vi "ECS-100X-FPGA1-EPTx.vi"() -> ()   [LabVIEW 2015, in "ECS-FPGA.lvlib"]
uses:
  ECS-FPGA.lvlib
  <vilib>/addons/Combustion Analysis System/FPGA/Controls/CAS - FPGA - Sample Data.ctl
  <vilib>/addons/Combustion Analysis System/FPGA/Controls/CAS - FPGA - EPT Data.ctl
  <vilib>/addons/Combustion Analysis System/FPGA/Controls/CAS - FPGA - Encoder Signals.ctl
  <vilib>/addons/Combustion Analysis System/FPGA/Controls/CAS - FPGA - Sample Control.ctl
  <vilib>/addons/Combustion Analysis System/FPGA/Controls/CAS - FPGA - Encoder Settings.ctl
  <vilib>/addons/Combustion Analysis System/FPGA/Controls/CAS - FPGA - EPT Control.ctl
  <vilib>/Powertrain Controls/Device Drivers/Engine Position Tracking/EPTx/RevA/FPGA/Controls/EPTxSupervisor.ctl
  <vilib>/Powertrain Controls/Device Drivers/Engine Position Tracking/EPTx/RevA/FPGA/Controls/EPTxConfig.ctl
  <vilib>/Powertrain Controls/Device Drivers/Engine Position Tracking/EPTx/RevA/FPGA/Controls/EPTxControl.ctl
  <vilib>/Powertrain Controls/Device Drivers/Engine Position Tracking/EPTx/RevA/FPGA/Controls/EPTxTooth.ctl
  <vilib>/Powertrain Controls/Device Drivers/Engine Position Tracking/EPTx/RevA/FPGA/Controls/EPTxEncoderConfig.ctl
  <vilib>/Powertrain Controls/Device Drivers/Engine Position Tracking/EPTx/RevA/FPGA/Controls/EPTxAAPControl.ctl
  <vilib>/Powertrain Controls/Device Drivers/Engine Position Tracking/EPTx/RevA/FPGA/Controls/EPTxFuelSparkControl.ctl
  <vilib>/Powertrain Controls/Device Drivers/FPGA Knock/RevA/FPGA/Controls/Knock Settings.ctl
  <vilib>/Powertrain Controls/Device Drivers/FPGA Knock/RevA/FPGA/Controls/EPTx Window.ctl
  <vilib>/Platform/TimedLoop/XDataNode/timing_clust.ctl
  <vilib>/Platform/TimedLoop/XDataNode/nitl_modes.ctl
  <vilib>/Platform/TimedLoop/XDataNode/wakeup.ctl
  <vilib>/Powertrain Controls/Device Drivers/Engine Position Tracking/EPTx/RevA/FPGA/Controls/EPTxSignals.ctl
  <vilib>/rvi/Emulation/niFpgaGetClockAttributes.vi
  <vilib>/rvi/Emulation/niFpgaSctlEmulationGetInTimedLoop.vi
  <vilib>/rvi/Emulation/niFpgaEmulationReportErrorSimple.vi
  <vilib>/rvi/eio/common/nirviEmuTemplateMethod_errors.vi
  <vilib>/rvi/Emulation/niFpgaCriticalErrorInLSC.vi
  <vilib>/rvi/Emulation/niFpgaProcessEmulError.vi
  <vilib>/eio/EIOMethodNode/EIOMethodNode.xnode
  <vilib>/eio/EIONode/EIONode.xnode
  <vilib>/LabVIEW Targets/FPGA/RIO/nicrio_985x_controls.llb/CAN_IO_Frame Cluster.ctl
  <vilib>/LabVIEW Targets/FPGA/RIO/nicrio_985x_controls.llb/CAN_IO_Frame Type.ctl
  <vilib>/Platform/TimedLoop/XDataNode/XDataNode.xnode
  <vilib>/Platform/TimedLoop/XDataNode/XDNodeRunTimeDep.lvlib
  <vilib>/Powertrain Controls/Device Drivers/Engine Position Tracking/EPTx/RevA/FPGA/EPTx - RevA - FPGA.lvlib
  <vilib>/Powertrain Controls/Device Drivers/FPGA Knock/RevA/FPGA/Knock - RevA - FPGA.lvlib
panel:
  in  "Knock.SensorIndexes":i32[](array[numeric])=[0, 0, 0, 0, 0, 0, 0, 0, 0, 0, 0, 0, 0, 0, 0, 0]
  out "Knock.Running":bool
  in  "Knock.Windows":cluster{"Index":fxp<+,4,4>, "EPT Windows":T1}
  in  "Knock.Settings":T2={"Sample Clock [Ticks]"=0, "Threshold"=0.0, "Coeff A"=[0.0, 0.0, 0.0, 0.0], "Coeff B"=[0.0, 0.0, 0.0, 0.0, 0.0, 0.0]}
  out "Knock.Results":bool[](array[boolean])
  out "Knock.Intensity":fxp<+,8,4>[](array[numeric]) format="%.6g"
  in  "O2-1.Control":T3
  out "O2-1.Data":T4
  in  "DI-1.PlsGen_Config_Channel3":T5
  in  "DI-1.PlsGen_Config_Channel2":T5
  in  "DI-1.PlsGen_Config_Channel1":T5
  in  "EPTx.Gate/Reset":u8=1
  in  "EPTx.EncoderZ":u8=1
  in  "EPTx.EncoderB":u8=1
  in  "EPTx.EncSignalSelect":bool
  in  "ESTTL-1.Sequences":T6(array[cluster])
  in  "ESTTL-1.Config":T7
  in  "PFI-1.FuelControl 4":T8
  in  "PFI-1.FuelControl 3":T8
  in  "PFI-1.FuelControl 2":T8
  in  "PFI-1.FuelControl 1":T8
  out "EPTx.Aux4CaptureCAD":fxp<+,18,11>
  out "EPTx.Aux3CaptureCAD":fxp<+,18,11>
  out "EPTx.Aux2CaptureCAD":fxp<+,18,11>
  out "EPTx.Aux1CaptureCAD":fxp<+,18,11>
  out "EPTx.Aux4EdgeCount":u8
  out "EPTx.Aux3EdgeCount":u8
  out "EPTx.Aux2EdgeCount":u8
  out "EPTx.Aux1EdgeCount":u8
  in  "EPTx.Aux4AngleCapture":T9
  in  "EPTx.Aux3AngleCapture":T9
  in  "EPTx.Aux2AngleCapture":T9
  in  "EPTx.Aux1AngleCapture":T9
  in  "EPTx.EncoderA":u8=1
  in  "EPTxEncoderConfig":T10
  out "EPTxTooth":T11
  in  "EPTxControl":T12
  in  "EPTxConfig":T13
  out "EPTxSupervisor":T14
  out "ADCombo-1.DigitalTriggers":u32
  in  "UserData.Data0":u32
  in  "UserData.Data1":u32
  in  "UserData.Data2":u32
  in  "UserData.Data3":u32
  in  "UserData.Period [ms]":u32=1
  in  "UserData.EnableFPGAData":bool
  in  "UserData.Data4":u32
  in  "UserData.Data5":u32
  in  "UserData.Data6":u32
  in  "UserData.Data7":u32
  in  "CAS-EPT Control":T15
  in  "CAS-Encoder Settings":T16
  in  "CAS-Sample Control":T17
  out "CAS-Encoder Signals":T18
  out "CAS-EPT Data":T19
  out "CAS-Sample Data":T20
  in  "CAS-Encoder Debug":bool
  out "CAS-Debug Overflow":bool
  out "Throttle-1.Data":T21 caption="ThrottleData"
  in  "Throttle-1.Control":T22 caption="ThrottleControl"
  out "ADCombo-1.VRHallData":T23 caption="VRHallData"
  in  "EPTx.Aux4":u8=2
  in  "EPTx.Aux2":u8=1
  out "DI-1.Data":T24 caption="DIData"
  in  "ADCombo-1.VRHallInvert":u8
  in  "ADCombo-1.VR1.Filt":u16
  in  "ADCombo-1.VR2.Filt":u16
  in  "ADCombo-1.Hall1.Filt":u16
  in  "ADCombo-1.Hall2.Filt":u16
  in  "9411-1.0.Filt":u16
  in  "9411-1.1.Filt":u16
  in  "9411-1.2.Filt":u16
  in  "9411-1.3.Filt":u16
  in  "9411-1.4.Filt":u16
  in  "9411-1.5.Filt":u16
  in  "9411-1.Invert":u8
  in  "9755-1.Sensor 1 Enable":bool
  in  "9755-1.RxID 1":u32=418385746 format="%08x"
  in  "9755-1.TxID":u32=419356416 format="%08x"
  in  "9755-1.CAN0 Restart":bool
  out "9755-1.NOxSensorData 1":T25={"NOx (bits)"=0, "O2 (bits)"=0, "Sensor Supply Status"=3, "Sensor Temperature Status"=12, "NOx Signal Status"=48, "O2 Signal Status"=192, "Heater Mode Status"=96, "Heater Circuit Status"=31, "NOx Circuit Status"=31, "O2 Circuit Status"=31, "NOx Sensor Module Present"=FALSE} {"Heater Mode Status" items=["AUTO MODE"=0, "HEATUP SLOPE 3 OR 4"=32, "HEATUP SLOPE 1 OR 2"=64, "HEATER OFF / PREHEAT"=96]; "O2 Circuit Status" items=["OPEN WIRE"=3, "SHORT CIRCUIT"=5, "NO ERROR"=31]; "NOx Circuit Status" items=["OPEN WIRE"=3, "SHORT CIRCUIT"=5, "NO ERROR"=31]; "Heater Circuit Status" items=["OPEN WIRE"=3, "SHORT CIRCUIT"=5, "NO ERROR"=31]; "Sensor Temperature Status" items=["NOT AT TEMPERATURE"=0, "AT TEMPERATURE"=4, "ERROR"=8, "NOT AVAILABLE"=12]; "O2 Signal Status" items=["NOT VALID"=0, "VALID"=64, "ERROR"=128, "NOT AVAILABLE"=192]; "NOx Signal Status" items=["NOT VALID"=0, "VALID"=16, "ERROR"=32, "NOT AVAILABLE"=48]; "Sensor Supply Status" items=["NOT IN RANGE", "SUPPLY IN RANGE", "ERROR", "NOT AVAILABLE"]}
  out "9755-1.RxID Actual":u32 format="%08x"
  in  "9755-1.Sensor 2 Enable":bool
  in  "9755-1.RxID 2":u32=418385489 format="%08x"
  out "9755-1.NOxSensorData 2":T25={"NOx (bits)"=0, "O2 (bits)"=0, "Sensor Supply Status"=3, "Sensor Temperature Status"=12, "NOx Signal Status"=48, "O2 Signal Status"=192, "Heater Mode Status"=96, "Heater Circuit Status"=31, "NOx Circuit Status"=31, "O2 Circuit Status"=31, "NOx Sensor Module Present"=FALSE} {"Heater Mode Status" items=["AUTO MODE"=0, "HEATUP SLOPE 3 OR 4"=32, "HEATUP SLOPE 1 OR 2"=64, "HEATER OFF / PREHEAT"=96]; "O2 Circuit Status" items=["OPEN WIRE"=3, "SHORT CIRCUIT"=5, "NO ERROR"=31]; "NOx Circuit Status" items=["OPEN WIRE"=3, "SHORT CIRCUIT"=5, "NO ERROR"=31]; "Heater Circuit Status" items=["OPEN WIRE"=3, "SHORT CIRCUIT"=5, "NO ERROR"=31]; "Sensor Temperature Status" items=["NOT AT TEMPERATURE"=0, "AT TEMPERATURE"=4, "ERROR"=8, "NOT AVAILABLE"=12]; "O2 Signal Status" items=["NOT VALID"=0, "VALID"=64, "ERROR"=128, "NOT AVAILABLE"=192]; "NOx Signal Status" items=["NOT VALID"=0, "VALID"=16, "ERROR"=32, "NOT AVAILABLE"=48]; "Sensor Supply Status" items=["NOT IN RANGE", "SUPPLY IN RANGE", "ERROR", "NOT AVAILABLE"]}
  in  "Power.TDK_Rly_Ctrl":bool
  in  "Power.12V_Rly_Ctrl":bool
  in  "Power.5V_Rly_Ctrl":bool
  out "ADCombo-1.ModulePresent":bool caption="ModulePresent"
  out "PFI-1.Data":T26 caption="PFIData"
  in  "PFI-1.IPhaseInterface":T27(array[cluster])=[{"IPhaseCurrent"=0, "IPhaseDuration"=0}, {"IPhaseCurrent"=0, "IPhaseDuration"=0}, {"IPhaseCurrent"=0, "IPhaseDuration"=0}, {"IPhaseCurrent"=0, "IPhaseDuration"=0}, {"IPhaseCurrent"=0, "IPhaseDuration"=0}, {"IPhaseCurrent"=0, "IPhaseDuration"=0}, {"IPhaseCurrent"=0, "IPhaseDuration"=0}, {"IPhaseCurrent"=0, "IPhaseDuration"=0}] caption="IPhaseInterface"
  in  "PFI-1.LowsidePWM":T28 caption="LowsidePWM"
  in  "PFI-1.Control":T29 caption="PFIControl"
  out "DI-1.ScopeData":T30 caption="DIScopeData"
  in  "DI-1.ScopeRead":bool caption="DIScopeRead"
  in  "DI-1.IPhaseInterface":T31(array[cluster]) caption="IPhaseInterface"
  in  "DI-1.Control":T32 caption="DIControl"
  in  "EPTx.Aux3":u8
  in  "EPTx.Primary":u8
  in  "EPTx.Aux1":u8
  out "ADCombo-1.Hall1.PPWData":T33
  out "ADCombo-1.Hall2.PPWData":T33
  out "ADCombo-1.VR2.PPWData":T33
  out "ADCombo-1.VR1.PPWData":T33
  out "9411-1.0.PPWData":T33
  out "9411-1.1.PPWData":T33
  out "9411-1.2.PPWData":T33
  out "9411-1.3.PPWData":T33
  out "9411-1.4.PPWData":T33
  out "9411-1.5.PPWData":T33
  out "9411-1.DigitalTriggers":u32
  out "ADCombo-1.AnalogData":T34 caption="AnalogData"
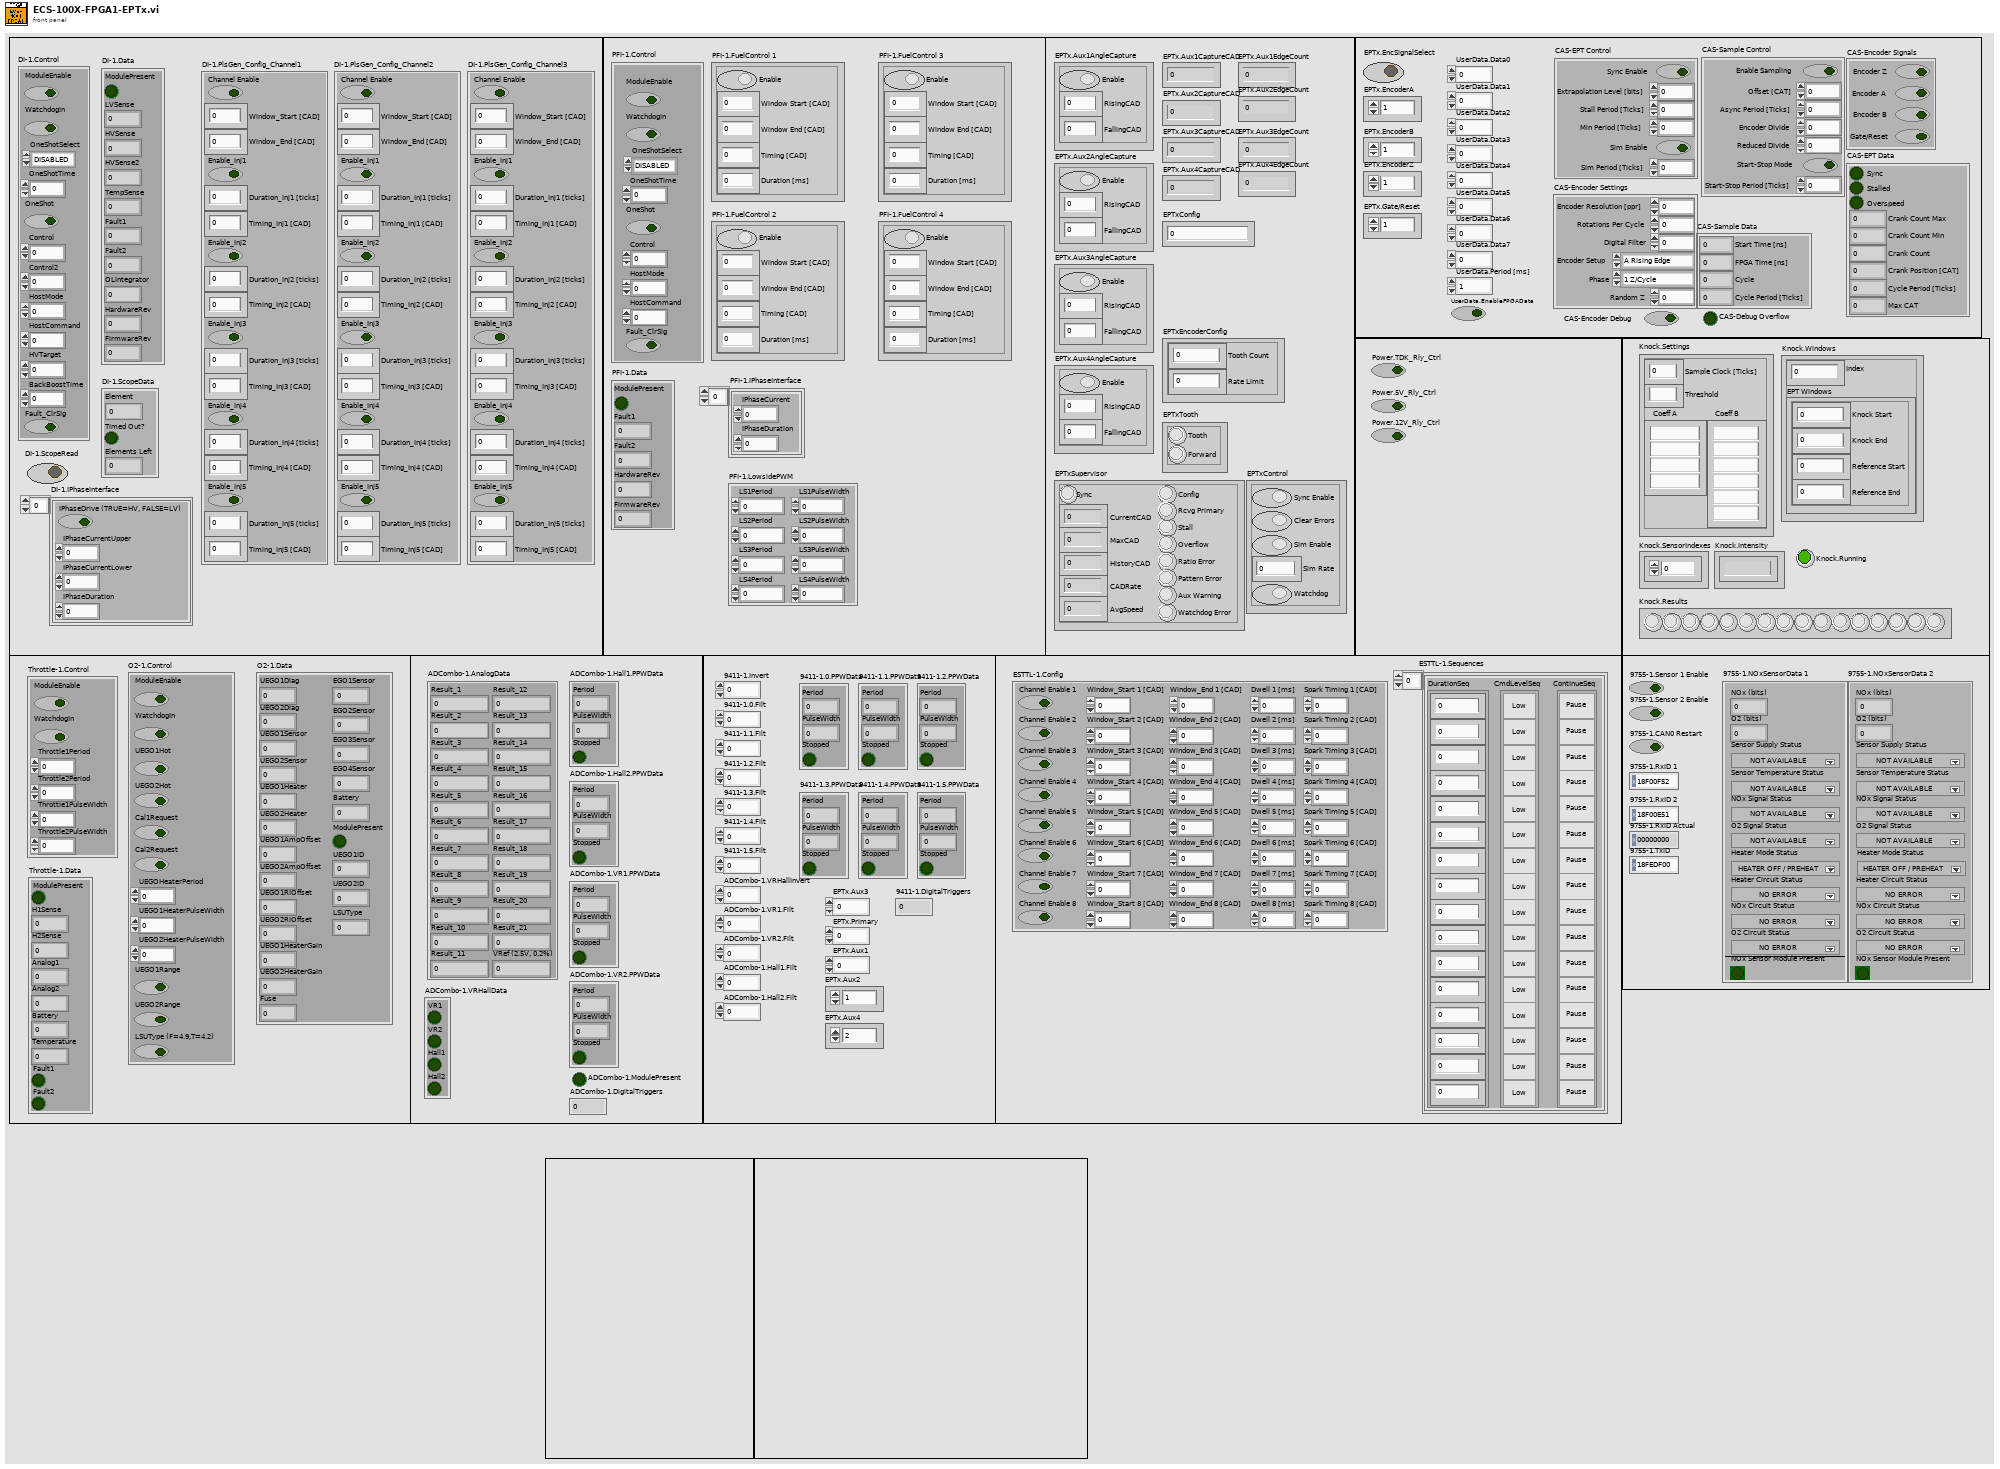
[diagram p1: front panel]
types:
  T1 = typedef "Knock - RevA - FPGA.lvlib/EPTx Window.ctl" = cluster{"Knock Start":fxp<+,18,11>, "Knock End":fxp<+,18,11>, "Reference Start":fxp<+,18,11>, "Reference End":fxp<+,18,11>}
  T2 = typedef "Knock - RevA - FPGA.lvlib/Knock Settings.ctl" = cluster{"Sample Clock [Ticks]":u16, "Threshold":fxp<+,10,4>, "Coeff A":fxp<+/-,16,2>[], "Coeff B":fxp<+/-,20,3>[]}
  T3 = cluster{"ModuleEnable":bool, "WatchdogIn":bool, "UEGO1Hot":bool, "UEGO2Hot":bool, "Cal1Request":bool, "Cal2Request":bool, "UEGOHeaterPeriod":u16, "UEGO1HeaterPulseWidth":u16, "UEGO2HeaterPulseWidth":u16, "UEGO1Range":bool, "UEGO2Range":bool, "LSUType (F=4.9,T=4.2)":bool}
  T4 = cluster{"UEGO1Diag":u8, "UEGO2Diag":u8, "UEGO1Sensor":u16, "UEGO2Sensor":u16, "UEGO1Heater":u16, "UEGO2Heater":u16, "UEGO1AmpOffset":u16, "UEGO2AmpOffset":u16, "UEGO1RIOffset":u16, "UEGO2RIOffset":u16, "UEGO1HeaterGain":u16, "UEGO2HeaterGain":u16, "Fuse":u16, "EGO1Sensor":u16, "EGO2Sensor":u16, "EGO3Sensor":u16, "EGO4Sensor":u16, "Battery":u16, "ModulePresent":bool, "UEGO1ID":u8, "UEGO2ID":u8, "LSUType":u8}
  T5 = cluster{"Channel Enable":bool, "Window_Start [CAD]":fxp<+,18,11>, "Window_End [CAD]":fxp<+,18,11>, "Enable_Inj1":bool, "Duration_Inj1 [ticks]":u32, "Timing_Inj1 [CAD]":fxp<+,18,11>, "Enable_Inj2":bool, "Duration_Inj2 [ticks]":u32, "Timing_Inj2 [CAD]":fxp<+,18,11>, "Enable_Inj3":bool, "Duration_Inj3 [ticks]":u32, "Timing_Inj3 [CAD]":fxp<+,18,11>, "Enable_Inj4":bool, "Duration_Inj4 [ticks]":u32, "Timing_Inj4 [CAD]":fxp<+,18,11>, "Enable_Inj5":bool, "Duration_Inj5 [ticks]":u32, "Timing_Inj5 [CAD]":fxp<+,18,11>}
  T6 = cluster{"DurationSeq":u32[], "CmdLevelSeq":bool[], "ContinueSeq":bool[]}[]
  T7 = cluster{"Channel Enable 1":bool, "Window_Start 1 [CAD]":fxp<+,18,11>, "Window_End 1 [CAD]":fxp<+,18,11>, "Dwell 1 [ms]":fxp<+/-,22,9>, "Spark Timing 1 [CAD]":fxp<+,18,11>, "Channel Enable 2":bool, "Window_Start 2 [CAD]":fxp<+,18,11>, "Window_End 2 [CAD]":fxp<+,18,11>, "Dwell 2 [ms]":fxp<+/-,22,9>, "Spark Timing 2 [CAD]":fxp<+,18,11>, "Channel Enable 3":bool, "Window_Start 3 [CAD]":fxp<+,18,11>, "Window_End 3 [CAD]":fxp<+,18,11>, "Dwell 3 [ms]":fxp<+/-,22,9>, "Spark Timing 3 [CAD]":fxp<+,18,11>, "Channel Enable 4":bool, "Window_Start 4 [CAD]":fxp<+,18,11>, "Window_End 4 [CAD]":fxp<+,18,11>, "Dwell 4 [ms]":fxp<+/-,22,9>, "Spark Timing 4 [CAD]":fxp<+,18,11>, "Channel Enable 5":bool, "Window_Start 5 [CAD]":fxp<+,18,11>, "Window_End 5 [CAD]":fxp<+,18,11>, "Dwell 5 [ms]":fxp<+/-,22,9>, "Spark Timing 5 [CAD]":fxp<+,18,11>, "Channel Enable 6":bool, "Window_Start 6 [CAD]":fxp<+,18,11>, "Window_End 6 [CAD]":fxp<+,18,11>, "Dwell 6 [ms]":fxp<+/-,22,9>, "Spark Timing 6 [CAD]":fxp<+,18,11>, "Channel Enable 7":bool, "Window_Start 7 [CAD]":fxp<+,18,11>, "Window_End 7 [CAD]":fxp<+,18,11>, "Dwell 7 [ms]":fxp<+/-,22,9>, "Spark Timing 7 [CAD]":fxp<+,18,11>, "Channel Enable 8":bool, "Window_Start 8 [CAD]":fxp<+,18,11>, "Window_End 8 [CAD]":fxp<+,18,11>, "Dwell 8 [ms]":fxp<+/-,22,9>, "Spark Timing 8 [CAD]":fxp<+,18,11>}
  T8 = typedef "EPTx - RevA - FPGA.lvlib/EPTxFuelSparkControl.ctl" = cluster{"Enable":bool, "Window Start [CAD]":fxp<+,18,11>, "Window End [CAD]":fxp<+,18,11>, "Timing [CAD]":fxp<+,18,11>, "Duration [ms]":fxp<+/-,22,9>}
  T9 = typedef "EPTx - RevA - FPGA.lvlib/EPTxAAPControl.ctl" = cluster{"Enable":bool, "RisingCAD":fxp<+,18,11>, "FallingCAD":fxp<+,18,11>}
  T10 = typedef "EPTx - RevA - FPGA.lvlib/EPTxEncoderConfig.ctl" = cluster{"Tooth Count":fxp<+,12,12>, "Rate Limit":fxp<+,12,12>}
  T11 = typedef "EPTx - RevA - FPGA.lvlib/EPTxTooth.ctl" = cluster{"Tooth":bool, "Forward":bool}
  T12 = typedef "EPTx - RevA - FPGA.lvlib/EPTxControl.ctl" = cluster{"Sync Enable":bool, "Clear Errors":bool, "Sim Enable":bool, "Sim Rate":fxp<+,24,6>, "Watchdog":bool}
  T13 = typedef "EPTx - RevA - FPGA.lvlib/EPTxConfig.ctl" = u64
  T14 = typedef "EPTx - RevA - FPGA.lvlib/EPTxSupervisor.ctl" = cluster{"Sync":bool, "CurrentCAD":fxp<+,18,11>, "MaxCAD":fxp<+,11,11>, "HistoryCAD":fxp<+,11,11>, "CADRate":fxp<+,22,8>, "AvgSpeed":fxp<+,17,15>, "Config":bool, "Rcvg Primary":bool, "Stall":bool, "Overflow":bool, "Ratio Error":bool, "Pattern Error":bool, "Aux Warning":bool, "Watchdog Error":bool}
  T15 = typedef "CAS - FPGA - EPT Control.ctl" = cluster{"Sync Enable":bool, "Extrapolation Level [bits]":u8, "Stall Period [Ticks]":u32, "Min Period [Ticks]":u32, "Sim Enable":bool, "Sim Period [Ticks]":u32}
  T16 = typedef "CAS - FPGA - Encoder Settings.ctl" = cluster{"Encoder Resolution [ppr]":u16, "Rotations Per Cycle":u8, "Digital Filter":u16, "Encoder Setup":enum8{"A Rising Edge", "A Any Edge", "A & B Any Edge"}, "Phase":enum8{"1 Z/Cycle", "Gate Z", "Random Z", "Reset Z"}, "Random Z":u8}
  T17 = typedef "CAS - FPGA - Sample Control.ctl" = cluster{"Enable Sampling":bool, "Offset [CAT]":i32, "Async Period [Ticks]":u32, "Encoder Divide":u8, "Reduced Divide":u8, "Start-Stop Mode":bool, "Start-Stop Period [Ticks]":u32}
  T18 = typedef "CAS - FPGA - Encoder Signals.ctl" = cluster{"Encoder Z":bool, "Encoder A":bool, "Encoder B":bool, "Gate/Reset":bool}
  T19 = typedef "CAS - FPGA - EPT Data.ctl" = cluster{"Sync":bool, "Stalled":bool, "Overspeed":bool, "Crank Count Max":u16, "Crank Count Min":u16, "Crank Count":u16, "Crank Position [CAT]":u16, "Cycle Period [Ticks]":u32, "Max CAT":u16}
  T20 = typedef "CAS - FPGA - Sample Data.ctl" = cluster{"Start Time [ns]":u64, "FPGA Time [ns]":u64, "Cycle":u32, "Cycle Period [Ticks]":u32}
  T21 = cluster{"ModulePresent":bool, "H1Sense":i16, "H2Sense":i16, "Analog1":i16, "Analog2":i16, "Battery":i16, "Temperature":i16, "Fault1":bool, "Fault2":bool}
  T22 = cluster{"ModuleEnable":bool, "WatchdogIn":bool, "Throttle1Period":u16, "Throttle2Period":u16, "Throttle1PulseWidth":i16, "Throttle2PulseWidth":i16}
  T23 = cluster{"VR1":bool, "VR2":bool, "Hall1":bool, "Hall2":bool}
  T24 = cluster{"ModulePresent":bool, "LVSense":u8, "HVSense":u8, "HVSense2":u8, "TempSense":i8, "Fault1":u8, "Fault2":u8, "OLIntegrator":u32, "HardwareRev":u8, "FirmwareRev":u8}
  T25 = cluster{"NOx (bits)":u16, "O2 (bits)":u16, "Sensor Supply Status":u8, "Sensor Temperature Status":u8, "NOx Signal Status":u8, "O2 Signal Status":u8, "Heater Mode Status":u8, "Heater Circuit Status":u8, "NOx Circuit Status":u8, "O2 Circuit Status":u8, "NOx Sensor Module Present":bool}
  T26 = cluster{"ModulePresent":bool, "Fault1":u8, "Fault2":u8, "HardwareRev":u8, "FirmwareRev":u8}
  T27 = cluster{"IPhaseCurrent":u16, "IPhaseDuration":u16}[]
  T28 = cluster{"LS1Period":u32, "LS1PulseWidth":u32, "LS2Period":u32, "LS2PulseWidth":u32, "LS3Period":u32, "LS3PulseWidth":u32, "LS4Period":u32, "LS4PulseWidth":u32}
  T29 = cluster{"ModuleEnable":bool, "WatchdogIn":bool, "OneShotSelect":enum8{"DISABLED", "PFI 1", "PFI 2", "PFI 3", "PFI 4"}, "OneShotTime":u32, "OneShot":bool, "Control":u16, "HostMode":u8, "HostCommand":u32, "Fault_ClrSig":bool}
  T30 = cluster{"Element":u32, "Timed Out?":bool, "Elements Left":u32}
  T31 = cluster{"IPhaseDrive (TRUE=HV, FALSE=LV)":bool, "IPhaseCurrentUpper":u16, "IPhaseCurrentLower":u16, "IPhaseDuration":u16}[]
  T32 = cluster{"ModuleEnable":bool, "WatchdogIn":bool, "OneShotSelect":enum8{"DISABLED", "CHAN 1", "CHAN 2", "CHAN 3"}, "OneShotTime":u32, "OneShot":bool, "Control":u8, "Control2":u8, "HostMode":u8, "HostCommand":u32, "HVTarget":u8, "BackBoostTime":u8, "Fault_ClrSig":bool}
  T33 = cluster{"Period":u32, "PulseWidth":u32, "Stopped":bool}
  T34 = cluster{"Result_1":u16, "Result_2":u16, "Result_3":u16, "Result_4":u16, "Result_5":u16, "Result_6":u16, "Result_7":u16, "Result_8":u16, "Result_9":u16, "Result_10":u16, "Result_11":u16, "Result_12":u16, "Result_13":u16, "Result_14":u16, "Result_15":u16, "Result_16":u16, "Result_17":u16, "Result_18":u16, "Result_19":u16, "Result_20":u16, "Result_21":u16, "VRef (2.5V, 0.2%)":u16}
  T35 = typedef "XDNodeRunTimeDep.lvlib/timing_clust.ctl" = cluster{"Expected End [f-1]":u64, "Actual End [f-1]":u64, "Finished Late? [f-1]":bool, "Expected End [i-1]":u64, "Actual End [i-1]":u64, "Finished Late? [i-1]":bool, "Expected Start [i]":u64, "Actual Start [i]":u64, "Expected Start [f]":u64, "Actual Start [f]":u64, "Source Name":string, "Structure Name":string, "Period":i64, "Deadline":i64, "Offset":i64, "Start":i64, "Priority":i32, "Timeout":i32, "Mode":T36, "Wakeup Reason":T37, "Error":errorcluster, "Source Type":string, "Secondary Source Type":string, "Global End Time":u64, "Global Start Time":u64, "Frame Duration":u64, "Iteration Duration":u64, "Assigned CPU":i32, "I/O Scan Engine Mode":u32}
  T36 = typedef "XDNodeRunTimeDep.lvlib/nitl_modes.ctl" = enum32{"No Change", "Process missed periods, maintain original phase", "Discard missed periods, maintain original phase", "Process missed periods, ignore original phase", "Discard missed periods, ignore original phase"}
  T37 = typedef "XDNodeRunTimeDep.lvlib/wakeup.ctl" = enum32{"Normal", "Aborted", "Asynchronous wakeup", "Timing source error", "Timed loop error", "Timeout"}
  T38 = typedef "EPTx - RevA - FPGA.lvlib/EPTxSignals.ctl" = cluster{"Primary":bool, "Aux 1":bool, "Aux 2":bool, "Aux 3":bool, "Aux 4":bool}
  T39 = typedef "EPTx - RevA - FPGA.lvlib/Encoder.ctl" = cluster{"Encoder A":bool, "Encoder B":bool, "Encoder Z":bool, "Encoder Cam":bool}
  T40 = typedef "CAS - FPGA - Trigger Signals.ctl" = cluster{"Start Trigger (TRIG0)":bool, "Sync Clock (TRIG1)":bool, "Async Clock (TRIG2)":bool, "Sync Data (TRIG3)":bool, "Async Data (TRIG4)":bool, "Reduced Resolution (TRIG5)":bool, "Reserved (TRIG6)":bool, "20MHz Clock (TRIG7)":bool}
  T41 = cluster{"CmdOut1":bool, "CmdOut2":bool, "CmdOut3":bool, "CmdOut4":bool, "CmdOut5":bool, "CmdOut6":bool, "CmdOut7":bool, "CmdOut8":bool}
  T42 = typedef "CAN_IO_Frame Cluster.ctl" = cluster{"timestamp high":u32, "timestamp low":u32, "identifier":u32, "type":T43, "info A":u8, "info B":u8, "data length":u8, "data":u8[]}
  T43 = typedef "CAN_IO_Frame Type.ctl" = enum8{"Data Frame", "Remote Frame", "(reserved)", "(reserved) ", "(reserved)  ", "(reserved)   ", "Bus Error", "Transceiver Fault"}
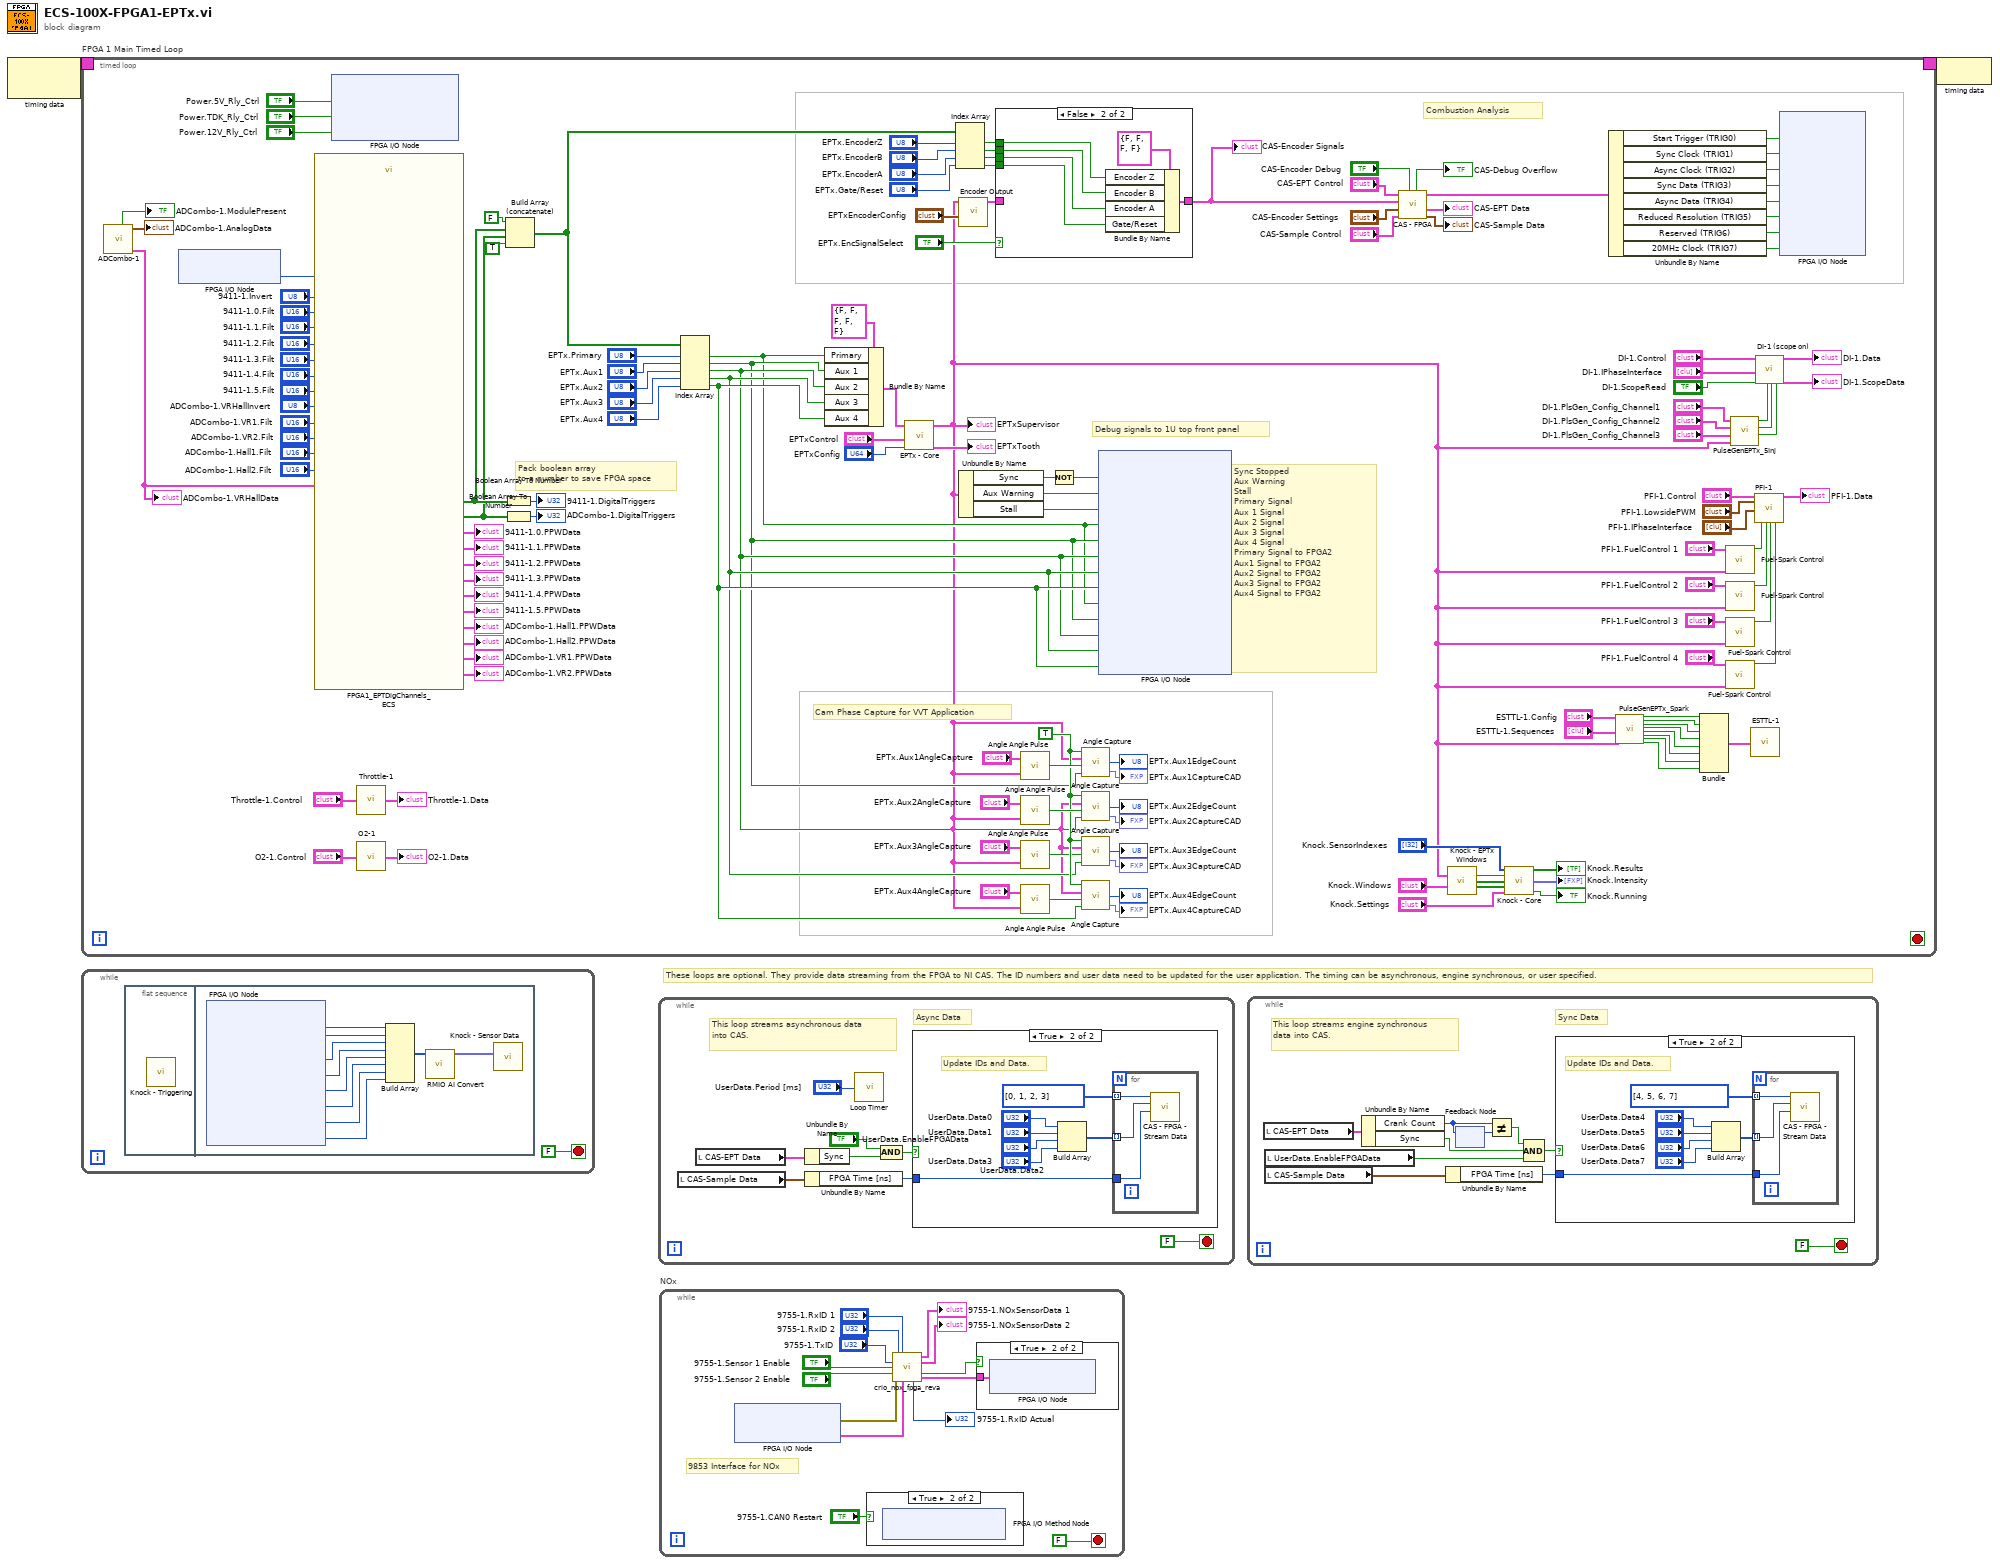
[diagram p0: block diagram]
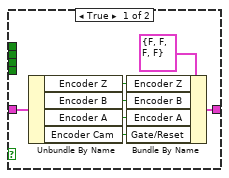
[diagram p6: hidden frame]
diagram:
  # "These loops are optional. They provide data streaming from the FPGA to NI CAS. The ID numbers and user data need to be updated for the user application. The timing can be asynchronous, engine synchronous, or user specified."
  n1 = node-c288() -> (w2:T35)  [unwired: 1 in]
  n2 = timed-loop "FPGA 1 Main Timed Loop" {
    timing: w2 -> [_]
    timing-out: [_] -> w1
    stop <- _ stop-if-true
    w53 = TRUE ("Enable")
    # "Pack boolean array\nto a number to save FPGA space"
    # "Cam Phase Capture for VVT Application"
    # "Combustion Analysis"
    # "Debug signals to 1U top front panel"
    # "Sync Stopped\nAux Warning\nStall\nPrimary Signal\nAux 1 Signal\nAux 2 Signal\nAux 3 Signal\nAux 4 Signal\nPrimary Signal to FPGA2\nAux1 Signal to FPGA2\nAux2 Signal to FPGA2\nAux3 Signal to FPGA2\nAux4 Signal to FPGA2"
    n3 = call "ADCombo-1"() -> ("ADCombo-1_VRHallData"=w150:T23, "ADCombo-1_AnalogData"=→"ADCombo-1.AnalogData":T34, "ADCombo-1_ModulePresent"=→"ADCombo-1.ModulePresent":bool)  [unwired: 5 in, 2 out]
    "ADCombo-1.VRHallData" <- w150
    n4 = xnode "FPGA I/O Node"() -> ("9411-1/DI5:0"=w147:u8)  [unwired: 1 in, 1 out]
    n5 = call "FPGA1_EPTDigChannels_ECS.vi"("NI9411-1.2.Filt"="9411-1.2.Filt", "NI9411-1.3.Filt"="9411-1.3.Filt", "NI9411-1.4.Filt"="9411-1.4.Filt", "NI9411-1.5.Filt"="9411-1.5.Filt", "ADCombo-1.VRHallData"=w150, "ADCombo-1.VR1.Filt"="ADCombo-1.VR1.Filt", "ADCombo-1.VR2.Filt"="ADCombo-1.VR2.Filt", "9411/DI5:0"=w147, "ADCombo-1.Hall1.Filt"="ADCombo-1.Hall1.Filt", "NI9411-1.1.Filt"="9411-1.1.Filt", "ADCombo-1.Hall2.Filt"="ADCombo-1.Hall2.Filt", "NI9411-1.Invert"="9411-1.Invert", "ADCombo-1.VRHallInvert"="ADCombo-1.VRHallInvert", "NI9411-1.0.Filt"="9411-1.0.Filt") -> ("9411-1.0.PPWData"=→"9411-1.0.PPWData":T33, "ADCombo-1.Hall2.PPWData"=→"ADCombo-1.Hall2.PPWData":T33, "9411-1.1.PPWData"=→"9411-1.1.PPWData":T33, "ADCombo-1.Hall1.PPWData"=→"ADCombo-1.Hall1.PPWData":T33, "9411-1.2.PPWData"=→"9411-1.2.PPWData":T33, "9411-1.3.PPWData"=→"9411-1.3.PPWData":T33, "9411-1.4.PPWData"=→"9411-1.4.PPWData":T33, "9411-1.5.PPWData"=→"9411-1.5.PPWData":T33, "9411-1.DigitalTriggers"=w78:bool[], "ADCombo-1.VR1.PPWData"=→"ADCombo-1.VR1.PPWData":T33, "ADCombo-1.VR2.PPWData"=→"ADCombo-1.VR2.PPWData":T33, "ADCombo-1.DigitalTriggers"=w77:bool[])  [unwired: 2 in]
    n6 = xnode "FPGA I/O Node"("Connector0/DIO5"="Power.5V_Rly_Ctrl", "Connector0/DIO6"="Power.TDK_Rly_Ctrl", "Connector0/DIO7"="Power.12V_Rly_Ctrl") -> ()  [unwired: 3 in, 3 out]
    n7 = call "Throttle-1"("Throttle-1_Control"="Throttle-1.Control") -> ("Throttle-1_Data"=→"Throttle-1.Data":T21)
    n8 = call "O2-1"("O2Control"="O2-1.Control") -> ("O2Data"=→"O2-1.Data":T4)
    n9 = Boolean Array To Number(Boolean array=w78) -> (number=→"9411-1.DigitalTriggers":u32)
    n10 = Boolean Array To Number(Boolean array=w77) -> (number=→"ADCombo-1.DigitalTriggers":u32)
    n11 = Build Array (concatenate)(FALSE, w78, w77, TRUE) -> (w63:bool[])
    n12 = Index Array(array=w63, index #1="EPTx.Primary", index #2="EPTx.Aux1", index #3="EPTx.Aux2", index #4="EPTx.Aux3", index #5="EPTx.Aux4") -> (element #1=w16:bool, element #2=w17:bool, element #3=w18:bool, element #4=w19:bool, element #5=w20:bool)
    n13 = Bundle By Name(cluster=T38 {"Primary"=FALSE, "Aux 1"=FALSE, "Aux 2"=FALSE, "Aux 3"=FALSE, "Aux 4"=FALSE} ("EPTxSignals"), "Primary"=w16, "Aux 1"=w17, "Aux 2"=w18, "Aux 3"=w19, "Aux 4"=w20) -> (w71:T38)
    n14 = call <vilib>:"EPTx - Core.vi"("EPTxConfig"="EPTxConfig", "EPTxControl"="EPTxControl", "EPTxSignals"=w71) -> ("EPTxTooth"=→"EPTxTooth":T11, "EPTxSupervisor"=w3:T14)  [unwired: 7 in]
    "EPTxSupervisor" <- w3
    n15 = Index Array(array=w63, index #1="EPTx.EncoderZ", index #2="EPTx.EncoderB", index #3="EPTx.EncoderA", index #4="EPTx.Gate/Reset") -> (element #1=w61:bool, element #2=w60:bool, element #3=w59:bool, element #4=w58:bool)
    n16 = call <vilib>:"Encoder Output.vi"("EPTxEncoderConfig"="EPTxEncoderConfig", "EPTxSupervisor"=w3) -> ("EncoderOutput"=w62:T39)  [unwired: 9 in]
    n17 = Unbundle By Name(w3) -> ("Sync"=w69:bool, "Aux Warning"=w67:bool, "Stall"=w15:bool)
    n18 = case shown="False" "EPTx.EncSignalSelect" {
      tunnel: [w156 w162] -> w65
      tunnel: w62 -> [w155 _]
      tunnel: w61 -> [_ w161]
      tunnel: w60 -> [_ w160]
      tunnel: w59 -> [_ w159]
      tunnel: w58 -> [_ w158]
      frame True {
        n19 = Unbundle By Name(w155) -> ("Encoder Z"=w151:bool, "Encoder B"=w152:bool, "Encoder A"=w153:bool, "Encoder Cam"=w154:bool)
        n20 = Bundle By Name(cluster=T18 {"Encoder Z"=FALSE, "Encoder A"=FALSE, "Encoder B"=FALSE, "Gate/Reset"=FALSE} ("Encoder Signal"), "Encoder Z"=w151, "Encoder B"=w152, "Encoder A"=w153, "Gate/Reset"=w154) -> (w156:T18)
      }
      frame False {
        n21 = Bundle By Name(cluster=T18 {"Encoder Z"=FALSE, "Encoder A"=FALSE, "Encoder B"=FALSE, "Gate/Reset"=FALSE} ("Encoder Signal"), "Encoder Z"=w161, "Encoder B"=w160, "Encoder A"=w159, "Gate/Reset"=w158) -> (w162:T18)
      }
    }
    "CAS-Encoder Signals" <- w65
    n22 = call <vilib>:"Angle Angle Pulse.vi"("EPTxSupervisor"=w3, "AAPControl"="EPTx.Aux1AngleCapture") -> ("AAP"=w55:bool)
    n23 = call <vilib>:"Angle Angle Pulse.vi"("EPTxSupervisor"=w3, "AAPControl"="EPTx.Aux2AngleCapture") -> ("AAP"=w54:bool)
    n24 = call <vilib>:"Angle Angle Pulse.vi"("EPTxSupervisor"=w3, "AAPControl"="EPTx.Aux3AngleCapture") -> ("AAP"=w31:bool)
    n25 = call <vilib>:"Angle Angle Pulse.vi"("EPTxSupervisor"=w3, "AAPControl"="EPTx.Aux4AngleCapture") -> ("AAP"=w28:bool)
    n26 = Not(x=w69) -> (.not. x?=w68:bool)
    n27 = call <vilib>:"Angle Capture.vi"("Capture"=w17, "OpWindow"=w55, "EPTxSupervisor"=w3, "Enable"=w53) -> ("CaptureCAD"=→"EPTx.Aux1CaptureCAD":fxp<+,18,11>, "CaptureCount"=→"EPTx.Aux1EdgeCount":u8)  [unwired: 1 out]
    n28 = call <vilib>:"Angle Capture.vi"("Capture"=w18, "OpWindow"=w54, "EPTxSupervisor"=w3, "Enable"=w53) -> ("CaptureCAD"=→"EPTx.Aux2CaptureCAD":fxp<+,18,11>, "CaptureCount"=→"EPTx.Aux2EdgeCount":u8)  [unwired: 1 out]
    n29 = call <vilib>:"Angle Capture.vi"("Capture"=w19, "OpWindow"=w31, "EPTxSupervisor"=w3, "Enable"=w53) -> ("CaptureCAD"=→"EPTx.Aux3CaptureCAD":fxp<+,18,11>, "CaptureCount"=→"EPTx.Aux3EdgeCount":u8)  [unwired: 1 out]
    n30 = call <vilib>:"Angle Capture.vi"("Capture"=w20, "OpWindow"=w28, "EPTxSupervisor"=w3, "Enable"=w53) -> ("CaptureCAD"=→"EPTx.Aux4CaptureCAD":fxp<+,18,11>, "CaptureCount"=→"EPTx.Aux4EdgeCount":u8)  [unwired: 1 out]
    n31 = xnode "FPGA I/O Node"("Connector0/DIO0"=w68, "Connector0/DIO1"=w67, "Connector0/DIO2"=w15, "Connector0/DIO3"=w16, "Connector0/DIO4"=w17, "Connector0/DIO8"=w18, "Connector0/DIO9"=w19, "Connector0/DIO10"=w20, "Connector0/DIO11"=w16, "Connector0/DIO12"=w17, "Connector0/DIO13"=w18, "Connector0/DIO14"=w19, "Connector0/DIO15"=w20) -> ()  [unwired: 13 in, 13 out]
    n32 = call <vilib>:"CAS - FPGA.vi"("Encoder Debug"="CAS-Encoder Debug", "Sample Control"="CAS-Sample Control", "Encoder Settings"="CAS-Encoder Settings", "Encoder Signal"=w65, "EPT Control"="CAS-EPT Control") -> ("Sample Data"=→"CAS-Sample Data":T20, "EPT Data"=→"CAS-EPT Data":T19, "Trigger"=w80:T40, "Debug Overflow"=→"CAS-Debug Overflow":bool)  [unwired: 2 in, 1 out]
    n33 = call <vilib>:"Knock - EPTx Windows.vi"("EPTxSupervisor"=w3, "EPTx Windows"="Knock.Windows") -> ("Sync"=w12:bool, "Knock Window"=w11:bool[], "Reference Window"=w4:bool[])  [unwired: 11 in]
    n34 = call <vilib>:"Knock - Core.vi"("Knock Sensor Indexes"="Knock.SensorIndexes", "Sync"=w12, "Knock Window"=w11, "Reference Window"=w4, "Knock Settings"="Knock.Settings") -> ("Knock State"=→"Knock.Results":bool[], "Knock Intensity"=→"Knock.Intensity":fxp<+,10,4>[], "Knock Running"=→"Knock.Running":bool)  [unwired: 8 in]
    n35 = Unbundle By Name(w80) -> ("Start Trigger (TRIG0)"=w110:bool, "Sync Clock (TRIG1)"=w109:bool, "Async Clock (TRIG2)"=w108:bool, "Sync Data (TRIG3)"=w107:bool, "Async Data (TRIG4)"=w106:bool, "Reduced Resolution (TRIG5)"=w105:bool, "Reserved (TRIG6)"=w104:bool, "20MHz Clock (TRIG7)"=w103:bool)
    n36 = call "PulseGenEPTx_Spark.vi"("Spark_Config"="ESTTL-1.Config", "Spark_Sequences"="ESTTL-1.Sequences", "EPTxSupervisor"=w3) -> ("CmdOut1"=w98:bool, "CmdOut2"=w97:bool, "CmdOut3"=w96:bool, "CmdOut4"=w95:bool, "CmdOut5"=w94:bool, "CmdOut6"=w93:bool, "CmdOut7"=w92:bool, "CmdOut8"=w91:bool)  [unwired: 17 in]
    n37 = Bundle("CmdOut1"=w98, "CmdOut2"=w97, "CmdOut3"=w96, "CmdOut4"=w95, "CmdOut5"=w94, "CmdOut6"=w93, "CmdOut7"=w92, "CmdOut8"=w91) -> (w90:T41)  [unwired: 1 out]
    n38 = call <vilib>:"Fuel-Spark Control.vi"("EPTxSupervisor"=w3, "Fuel-Spark Control"="PFI-1.FuelControl 1") -> ("Fuel-Spark Command"=w38:bool)  [unwired: 9 in]
    n39 = call <vilib>:"Fuel-Spark Control.vi"("EPTxSupervisor"=w3, "Fuel-Spark Control"="PFI-1.FuelControl 2") -> ("Fuel-Spark Command"=w39:bool)  [unwired: 9 in]
    n40 = call <vilib>:"Fuel-Spark Control.vi"("EPTxSupervisor"=w3, "Fuel-Spark Control"="PFI-1.FuelControl 3") -> ("Fuel-Spark Command"=w40:bool)  [unwired: 9 in]
    n41 = call <vilib>:"Fuel-Spark Control.vi"("EPTxSupervisor"=w3, "Fuel-Spark Control"="PFI-1.FuelControl 4") -> ("Fuel-Spark Command"=w41:bool)  [unwired: 9 in]
    n42 = call "PulseGenEPTx_5Inj.vi"("EPTxSupervisor"=w3, "Inj_Config_Channel3"="DI-1.PlsGen_Config_Channel3", "Inj_Config_Channel2"="DI-1.PlsGen_Config_Channel2", "Inj_Config_Channel1"="DI-1.PlsGen_Config_Channel1") -> ("CmdOut3"=w46:bool, "CmdOut2"=w47:bool, "CmdOut1"=w48:bool)  [unwired: 3 in]
    n43 = call "ESTTL-1"("ESTTL-1_ESTTLChan"=w90) -> ()  [unwired: 1 out]
    n44 = call "PFI-1"("PFI-1_Control"="PFI-1.Control", "PFI-1_LowsidePWM"="PFI-1.LowsidePWM", "PFI-1_IPhaseInterface"="PFI-1.IPhaseInterface", "PFI1Cmd"=w38, "PFI2Cmd"=w39, "PFI3Cmd"=w40, "PFI4Cmd"=w41) -> ("PFI-1_Data"=→"PFI-1.Data":T26)  [unwired: 11 in, 1 out]
    n45 = call "DI-1 (scope on)"("DI-1_Control"="DI-1.Control", "DI-1_IPhaseInterface"="DI-1.IPhaseInterface", "DI-1_ScopeRead"="DI-1.ScopeRead", "DI1Cmd"=w48, "DI2Cmd"=w47, "DI3Cmd"=w46) -> ("DI-1_Data"=→"DI-1.Data":T24, "DI-1_ScopeData"=→"DI-1.ScopeData":T30)  [unwired: 11 in, 1 out]
    n46 = xnode "FPGA I/O Node"("PXI_Trig0"=w110, "PXI_Trig1"=w109, "PXI_Trig2"=w108, "PXI_Trig3"=w107, "PXI_Trig4"=w106, "PXI_Trig5"=w105, "PXI_Trig6"=w104, "PXI_Trig7"=w103) -> ()  [unwired: 8 in, 8 out]
  }
  n47 = while {
    stop <- FALSE stop-if-true
    n48 = flat-sequence {
      frame #0 {
        n49 = call <vilib>:"Knock - Triggering.vi"() -> ()  [unwired: 12 in]
      }
      frame #1 {
        n50 = xnode "FPGA I/O Node"() -> ("Connector0/AI0"=w176:i16, "Connector0/AI1"=w175:i16, "Connector0/AI2"=w174:i16, "Connector0/AI3"=w173:i16, "Connector0/AI4"=w171:i16, "Connector0/AI5"=w170:i16, "Connector0/AI6"=w169:i16, "Connector0/AI7"=w168:i16)  [unwired: 8 in, 8 out]
        n51 = Build Array(w176, w175, w174, w173, w171, w170, w169, w168) -> (w172:i16[])
        n52 = call "RMIO AI Convert.vi"("AI [hexbits]"=w172) -> ("AI [V]"=w167:fxp<+/-,20,5>[])  [unwired: 10 in]
        n53 = call <vilib>:"Knock - Sensor Data.vi"("Sensor Data"=w167) -> ()  [unwired: 11 in]
      }
    }
  }
  n54 = while {
    stop <- FALSE stop-if-true
    # "This loop streams asynchronous data into CAS."
    # "Async Data"
    n55 = local read "CAS-Sample Data"() -> (w178:T20)
    n56 = local read "CAS-EPT Data"() -> (w180:T19)
    n57 = Unbundle By Name(w180) -> ("Sync"=w179:bool)
    n58 = Unbundle By Name(w178) -> ("FPGA Time [ns]"=w177:u64)
    n59 = call "Loop Timer"("Count(mSec)"="UserData.Period [ms]") -> ()  [unwired: 1 out]
    n60 = Compound Arithmetic op=AND("UserData.EnableFPGAData", w179) -> (w182:bool)
    n61 = case shown="True" w182 {
      tunnel: w177 -> [_ w185]
      frame False {
      }
      frame True {
        # "Update IDs and Data."
        n62 = Build Array("UserData.Data0", "UserData.Data1", "UserData.Data2", "UserData.Data3") -> (w187:u32[])
        n63 = for {
          tunnel: w185 -> [w192]
          tunnel: w187 -> [w194] mode=indexing
          tunnel: u64[] [0, 1, 2, 3] ("appended array") -> [w193] mode=indexing
          n64 = call <vilib>:"CAS - FPGA - Stream Data.vi"("FPGA Timer [ns]"=w192, "Data"=w194, "ID"=w193) -> ()  [unwired: 9 in]
        }
      }
    }
  }
  n65 = while "NOx" {
    stop <- FALSE stop-if-true
    # "9853 Interface for NOx"
    n66 = xnode "FPGA I/O Node"() -> ("error out"=w207:errorcluster, "9853-1/CAN0"=w206:T42)  [unwired: 2 in, 1 out]
    n67 = case shown="True" "9755-1.CAN0 Restart" {
      frame False {
      }
      frame True {
        n68 = xnode "FPGA I/O Method Node"() -> ()  [unwired: 1 in, 1 out]
      }
    }
    n69 = call <vilib>:"crio_nox_fpga_reva.vi"("RxID 2"="9755-1.RxID 2", "RxID 1"="9755-1.RxID 1", "TxID"="9755-1.TxID", "Sensor1Enable"="9755-1.Sensor 1 Enable", "Sensor2Enable"="9755-1.Sensor 2 Enable", "CAN Error In"=w207, "CAN Data In"=w206) -> ("NOxSensorData 1"=→"9755-1.NOxSensorData 1":T25, "NOxSensorData 2"=→"9755-1.NOxSensorData 2":T25, "Update CAN Out"=w204:bool, "RxIDActual"=→"9755-1.RxID Actual":u32, "CAN Data Out"=w203:T42)  [unwired: 4 in]
    n70 = case shown="True" w204 {
      tunnel: w203 -> [_ w209]
      frame False {
      }
      frame True {
        n71 = xnode "FPGA I/O Node"("9853-1/CAN0"=w209) -> ()  [unwired: 1 in, 1 out]
      }
    }
  }
  n72 = while {
    stop <- FALSE stop-if-true
    # "This loop streams engine synchronous data into CAS."
    # "Sync Data"
    n73 = local read "CAS-EPT Data"() -> (w212:T19)
    n74 = local read "UserData.EnableFPGAData"() -> (w215:bool)
    n75 = local read "CAS-Sample Data"() -> (w214:T20)
    n76 = Unbundle By Name(w212) -> ("Crank Count"=w211:u16, "Sync"=w210:bool)
    n77 = Unbundle By Name(w214) -> ("FPGA Time [ns]"=w213:u64)
    n78 = feedback-in #1(w211) -> ()
    n79 = feedback #1() -> (w217:u16)  [unwired: 1 out]
    n80 = Not Equal?(x=w211, y=w217) -> (x != y?=w216:bool)
    n81 = Compound Arithmetic op=AND(w216, w210, w215) -> (w218:bool)
    n82 = case shown="True" w218 {
      tunnel: w213 -> [_ w220]
      frame False {
      }
      frame True {
        # "Update IDs and Data."
        n83 = Build Array("UserData.Data4", "UserData.Data5", "UserData.Data6", "UserData.Data7") -> (w222:u32[])
        n84 = for {
          tunnel: w220 -> [w227]
          tunnel: w222 -> [w229] mode=indexing
          tunnel: u64[] [4, 5, 6, 7] ("appended array") -> [w228] mode=indexing
          n85 = call <vilib>:"CAS - FPGA - Stream Data.vi"("FPGA Timer [ns]"=w227, "Data"=w229, "ID"=w228) -> ()  [unwired: 9 in]
        }
      }
    }
  }
  n86 = node-c288(w1) -> ()
